vi "Solve Linear Eqs (General).vi"   [LabVIEW 2017, in "NI_AALPro.lvlib"]
uses:
  <vilib>/Analysis/NI_AALPro.lvlib
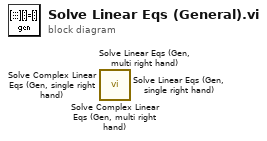
[diagram p0: block diagram]
diagram:
  n1 = call <vilib>:"Solve Complex Linear Eqs (Gen, multi right hand).vi"() -> ()  [unwired: 10 in, 2 out]
  n2 = call <vilib>:"Solve Linear Eqs (Gen, multi right hand).vi"() -> ()  [unwired: 10 in, 2 out]
  n3 = call <vilib>:"Solve Complex Linear Eqs (Gen, single right hand).vi"() -> ()  [unwired: 10 in, 2 out]
  n4 = call <vilib>:"Solve Linear Eqs (Gen, single right hand).vi"() -> ()  [unwired: 10 in, 2 out]
